vi "NHRDCPower.vi"() -> ()   [LabVIEW 2018, in "Visualization.lvlib" / "VisualizeAcPwr.lvclass"]
doc: "This VI listens for any measurement data associated with the provided PluginName and displays it to the user for analysis. The display is only suitable for data coming from the RoomAlert Plugin."
uses:
  VisualizeAcPwr.lvclass
  ChromaPowerSupply/Loop Parameters.ctl
  VisualizeBase/VisualizeBase_class/SubVIs/VisualizationOptions.ctl
  <vilib>/Utility/miscctls.llb/LVRectTypeDef.ctl
  AcPwr/AcPwrPlugins/NHRDCPowerClass/TypeDefs/Device(s)Settings.ctl
  AcPwr/AcPwrPlugins/NHRDCPowerClass/TypeDefs/Modules.ctl
  AcPwr/AcPwrPlugins/NHRDCPowerClass/TypeDefs/Measurements.ctl
  AcPwr/AcPwrShared/clMeasurmentData.ctl
  AcPwr/AcPwrPlugins/AcPwrBaseClass/TypeDefs/SetParameterInputs.ctl
  <vilib>/event_ctls.llb/usereventprio.ctl
  VisualizeBase/VisualizeBase_class/Requests/VisUserEventType.ctl
  <vilib>/Utility/error.llb/Error Cluster From Error Code.vi
  <vilib>/ErrorRing/Error Ring.xnode
  <userlib>/NIST/NISTErrorLib/NISTErrorLib.lvlib
  VisualizeBase/VisualizeBase_class/VisualizeBase.lvclass
  TestClass/Test.lvclass
  Sensor/VisualizeSensor.lvclass
  StatusAndLog/VisualizeStatus.lvclass
  AcPwr/AcPwrShared/AcPwrShared.lvlib
  AcPwr/AcPwrModule/AcPwrModule.lvlib
  AcPwr/AcPwrPlugins/AcPwrPlugins.lvlib
  AcPwr/AcPwrPlugins/AcPwrBaseClass/AcPwrBase.lvclass
  AcPwr/AcPwrPlugins/NHRDCPowerClass/NHRDCPower.lvclass
panel:
  out "Chart#":i32
  out "MeasChannels":string[](array[string])
  out "Writetime":u32 caption="Sample Write Time(ms)"
  out "ExitHelperLoops?":bool
  in  "Display":enum16{"Raw Data", "Voltage Vs Current"}(ring)
  in  "btnPause":bool
  in  "INIFilePath":path
  in  "ModuleID":i32
  in  "Log Data":bool=TRUE
  in  "btnStop":bool
  in  "btnReset":bool
  in  "btnClearTest":bool
  in  "btnStopModule":bool
  out "XY Graph":cluster{dbl[], dbl[]}(graph)
  out "Chart":waveform(dbl)[](graph)=[{"t0"=timestamp(3657200531.6397257 s since 1904-01-01), "dt"=1.0, "Y"=[46.19]}, {"t0"=timestamp(3657200531.6397257 s since 1904-01-01), "dt"=1.0, "Y"=[2.0]}, {"t0"=timestamp(3657200531.6397257 s since 1904-01-01), "dt"=1.0, "Y"=[60.0]}]
  in  "Power":bool
  in  "Power (W)":dbl
  in  "btnP_enable":bool
  in  "btnR_enable":bool
  in  "Resistance":bool
  in  "Resistance (Ohm)":dbl
  in  "btnI_enable":bool
  in  "Current":bool
  in  "Current (A)":dbl
  in  "btnV_Enable":bool
  in  "Voltage":bool
  in  "Voltage (V)":dbl
  in  "btnStopParameterLoop":bool
  in  "btnRunParamLoop":bool
  in  "Loop Parameters":T1={"Parameter"=enum."Voltage", "Start Value"=5.0, "Increment"=1.0, "Interval (s)"=3.0, "# Iterations"=6, "End Value"=10.0} {"# Iterations" min=1; "Increment" format="%#.4f"}
  out "ErrorArray":errorcluster[](array[cluster])
  out "Incorrect DataType?":bool
  out "String Results":string
  in  "PluginName":string="Sensor.RoomAlert1"
  # "Set Parameter"
  # "Parameter Looping"
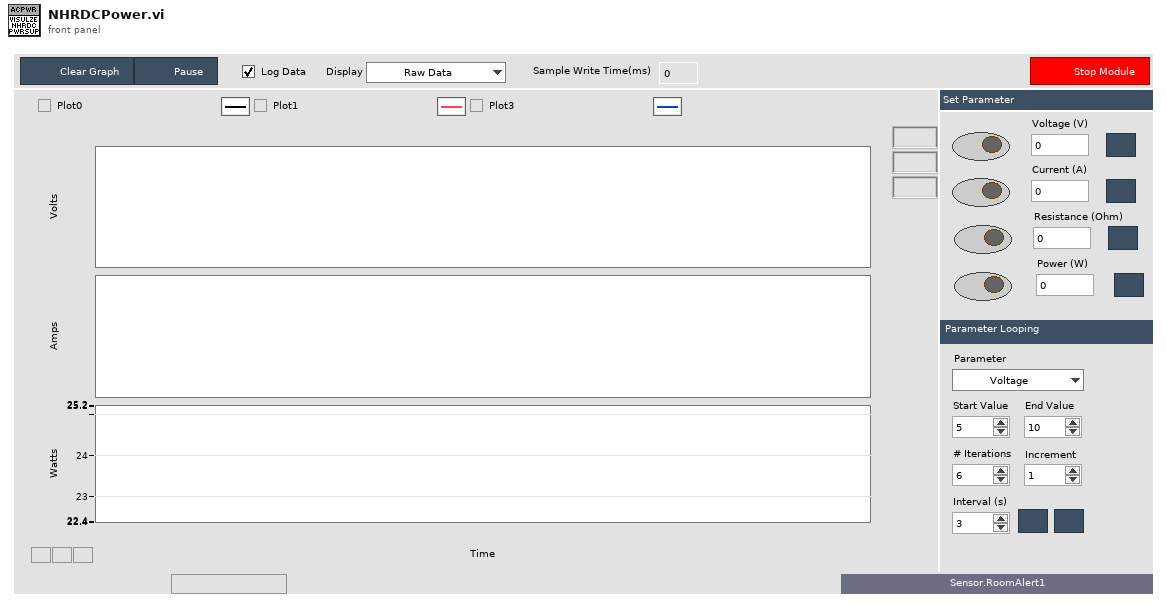
[diagram p1: front panel]
types:
  T1 = typedef "Loop Parameters.ctl" = cluster{"Parameter":enum16{"Voltage", "Current", "Power", "Resistance"}, "Start Value":dbl, "Increment":dbl, "Interval (s)":dbl, "# Iterations":u32, "End Value":dbl}
  T2 = typedef "Visualization.lvlib/VisualizeBase.lvclass/VisualizationOptions.ctl" = cluster{"PauseAtStartup":bool, "LogData":bool, "LaunchInSubPanel":bool, "FPMonitor":u16, "FPWindowBounds":T3, "MonitorBounds":cluster{"Left":i16, "Top":i16, "Right":i16, "Bottom":i16}, "MeasIndices":i32[]}
  T3 = typedef "LVRectTypeDef.ctl" = cluster{"Left":i16, "Top":i16, "Right":i16, "Bottom":i16}
  T4 = enum16{"open", "open or create", "create or replace", "create", "open (read-only)"}
  T5 = typedef "Visualization.lvlib/VisualizeBase.lvclass/VisRequestEvents.ctl" = cluster{"StopRequest":refnum<user-event>, "ResetRequest":refnum<user-event>, "FP Pop In or Out":refnum<user-event>}
  T6 = typedef "AcPwrShared.lvlib/AcPwrBroadcastEvents.ctl" = cluster{"DidInit":refnum<user-event>, "StatusUpdate":refnum<user-event>, "ErrorReport":refnum<user-event>, "DidStop":refnum<user-event>, "PathToINI":refnum<user-event>, "Measurements":refnum<user-event>, "LoadConfigFile":refnum<user-event>, "GetSettings":refnum<user-event>, "SetSettings":refnum<user-event>, "GetType&ID":refnum<user-event>, "GotSettings":refnum<user-event>, "GotSettingsLV":refnum<user-event>, "ParameterSet":refnum<user-event>}
  T7 = typedef "Visualization.lvlib/VisualizeBase.lvclass/VisFrmWrkBroadcastEvents.ctl" = cluster{"StatusUpdate":refnum<user-event>, "DidStop":refnum<user-event>, "NewModuleLoaded":refnum<user-event>, "StopVisualization":refnum<user-event>}
  T8 = typedef "AcPwrPlugins.lvlib/NHRDCPower.lvclass/Device(s)Settings.ctl" = cluster{"MeasName":string, "Modules":T9}
  T9 = typedef "AcPwrPlugins.lvlib/NHRDCPower.lvclass/Modules.ctl" = cluster{"Handle":string, "Name":string, "id query (Yes)":bool, "reset device (Yes)":bool, "Connected":bool, "Initial Battery Detect Voltage (0)":dbl, "SafetySettings":cluster{"SetWatchDog?":bool, "Voltage (V)":dbl, "Current (A)":dbl, "Power (W)":dbl, "Voltage Delay (s)":dbl, "Current Delay (s)":dbl, "Power Delay (s)":dbl}, "Options String":string, "Aperture Time (s)":dbl, "operating state (Off)":i32, "OutputSettings":cluster{"Voltage (V)":dbl, "Current (A)":dbl, "Resistance (Ohms)":dbl, "Power (W)":dbl, "Enable Voltage":bool, "Enable Current":bool, "Enable Resistance":bool, "Enable Power":bool, "Macro After Step Delay  (s)":dbl, "Wait Value (V, A, W)":dbl, "Enable Wait":bool, "Wait on Value":i32}[], "SlewRate":cluster{"Set Voltage Rate V/S":dbl, "Set Current Rate A/S":dbl, "Set Resistance Rate R/S":dbl, "Set Power Rate W/S":dbl}, "Macro":cluster{"Save Macro?":bool, "Load Macro From File?":bool, "Run Macro Continuously?":bool, "Use Macros?":bool, "Load Macro File Path":string, "Save Macro File Path":string}, "Regulation Gain (1=100%)":dbl, "UpdatingOntheFly":bool}[]
  T10 = typedef "AcPwrPlugins.lvlib/NHRDCPower.lvclass/Measurements.ctl" = cluster{"Handle":string, "Name":string, "Enabled":bool, "Measurement Value":sgl, "Measurement Type":enum16{"Power", "Current", "Voltage"}}[]
  T11 = typedef "AcPwrShared.lvlib/clMeasurmentData.ctl" = cluster{"MeasName":string, "XML Data":string, "WaveformData":waveform(dbl)[]}
  T12 = typedef "AcPwrPlugins.lvlib/AcPwrBase.lvclass/SetParameterInputs.ctl" = cluster{"Type":string, "Parameter":string, "Phase":i32, "Value":dbl, "Command":string, "Time Stamp":timestamp}
  T13 = typedef "Visualization.lvlib/VisualizeBase.lvclass/VisUserEventType.ctl" = cluster{"BusIndex":i8, "Data":variant}
  T14 = typedef "usereventprio.ctl" = enum32{"high priority", "normal priority"}
  T15 = cluster{"Handle":string, "Name":string, "id query (Yes)":bool, "reset device (Yes)":bool, "Connected":bool, "Initial Battery Detect Voltage (0)":dbl, "SafetySettings":cluster{"SetWatchDog?":bool, "Voltage (V)":dbl, "Current (A)":dbl, "Power (W)":dbl, "Voltage Delay (s)":dbl, "Current Delay (s)":dbl, "Power Delay (s)":dbl}, "Options String":string, "Aperture Time (s)":dbl, "operating state (Off)":i32, "OutputSettings":cluster{"Voltage (V)":dbl, "Current (A)":dbl, "Resistance (Ohms)":dbl, "Power (W)":dbl, "Enable Voltage":bool, "Enable Current":bool, "Enable Resistance":bool, "Enable Power":bool, "Macro After Step Delay  (s)":dbl, "Wait Value (V, A, W)":dbl, "Enable Wait":bool, "Wait on Value":i32}[], "SlewRate":cluster{"Set Voltage Rate V/S":dbl, "Set Current Rate A/S":dbl, "Set Resistance Rate R/S":dbl, "Set Power Rate W/S":dbl}, "Macro":cluster{"Save Macro?":bool, "Load Macro From File?":bool, "Run Macro Continuously?":bool, "Use Macros?":bool, "Load Macro File Path":string, "Save Macro File Path":string}, "Regulation Gain (1=100%)":dbl, "UpdatingOntheFly":bool}
  T16 = cluster{"Voltage (V)":dbl, "Current (A)":dbl, "Resistance (Ohms)":dbl, "Power (W)":dbl, "Enable Voltage":bool, "Enable Current":bool, "Enable Resistance":bool, "Enable Power":bool, "Macro After Step Delay  (s)":dbl, "Wait Value (V, A, W)":dbl, "Enable Wait":bool, "Wait on Value":i32}[]
  T17 = cluster{"Voltage (V)":dbl, "Current (A)":dbl, "Resistance (Ohms)":dbl, "Power (W)":dbl, "Enable Voltage":bool, "Enable Current":bool, "Enable Resistance":bool, "Enable Power":bool, "Macro After Step Delay  (s)":dbl, "Wait Value (V, A, W)":dbl, "Enable Wait":bool, "Wait on Value":i32}
  T18 = cluster{"Voltage (V)":dbl, "Current (A)":dbl, "Resistance (Ohm)":dbl, "Power (W)":dbl, "btnV_Enable":bool, "btnI_enable":bool, "btnR_enable":bool, "btnP_enable":bool}
  T19 = typedef "sizeaction.ctl" = enum32{"Minimized", "Maximized", "Resized"}
  T20 = typedef "LVPoint32TypeDef.ctl" = cluster{"Horizontal":i32, "Vertical":i32}
  T21 = enum16{"Voltage", "Current", "Power", "Resistance"}
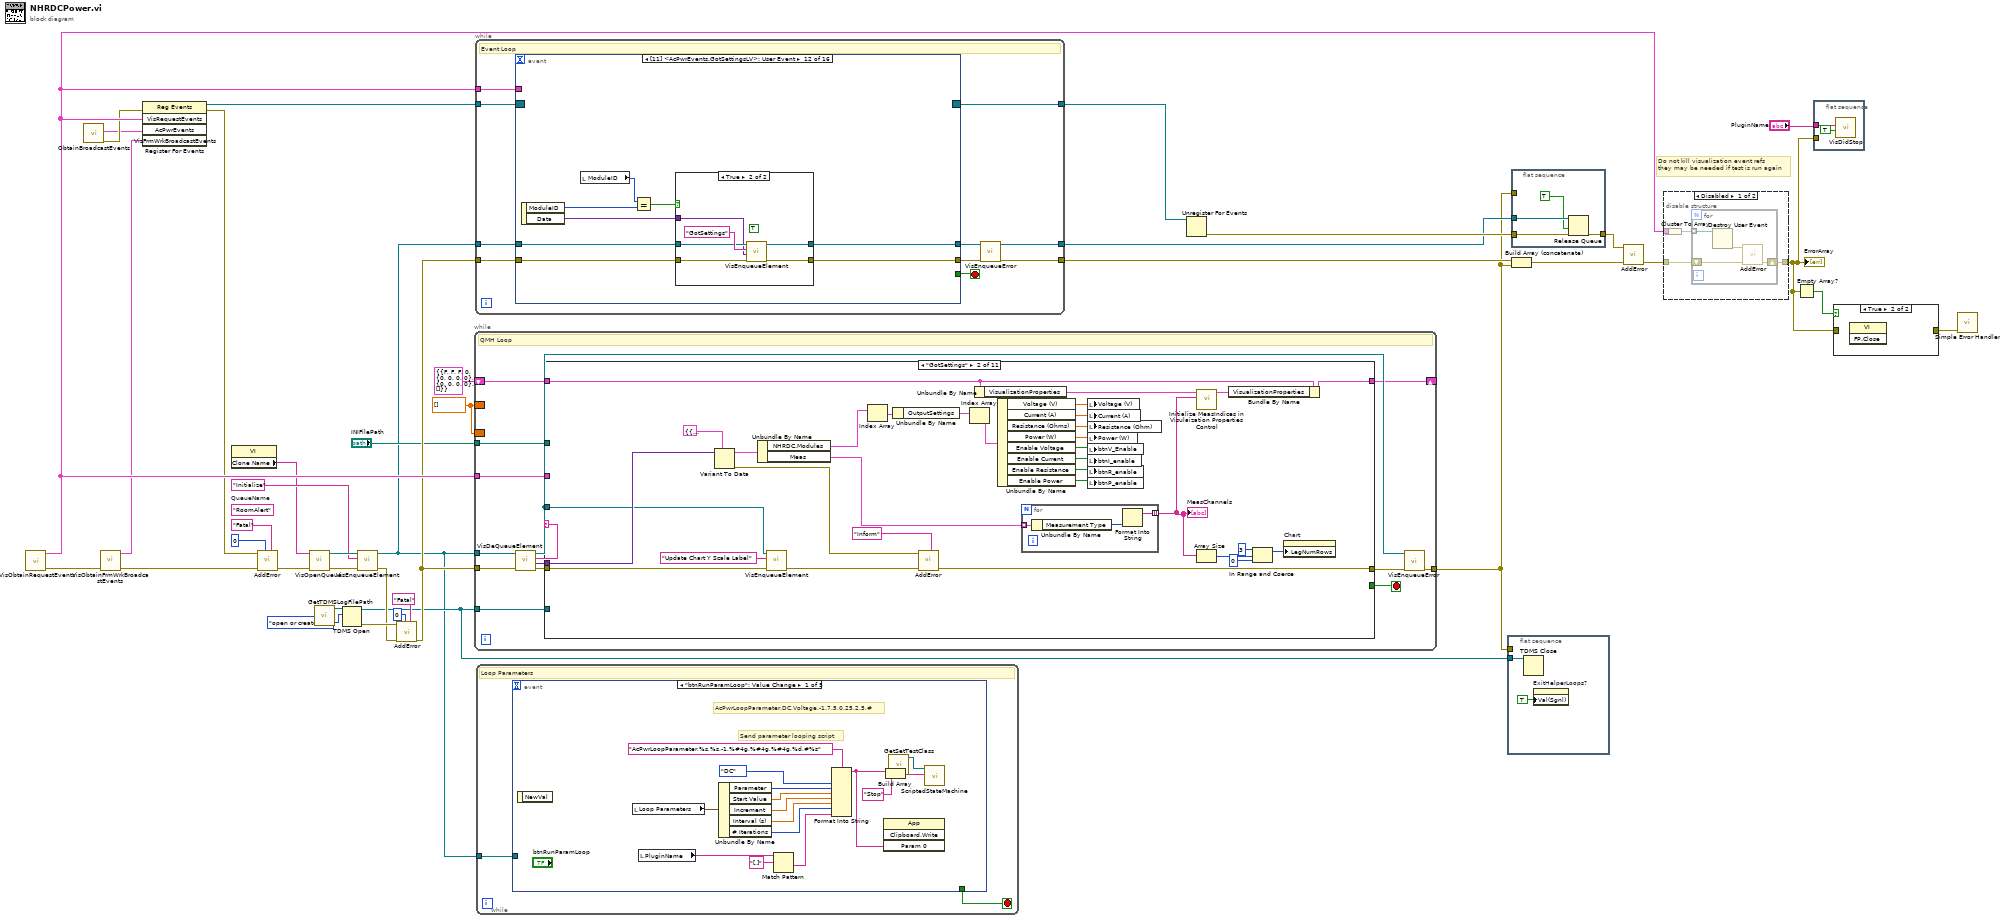
[diagram p0: block diagram]
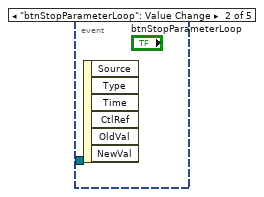
[diagram p2: hidden frame]
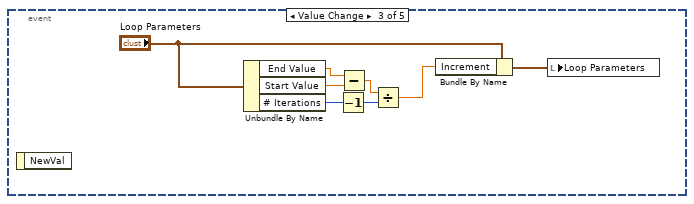
[diagram p3: hidden frame]
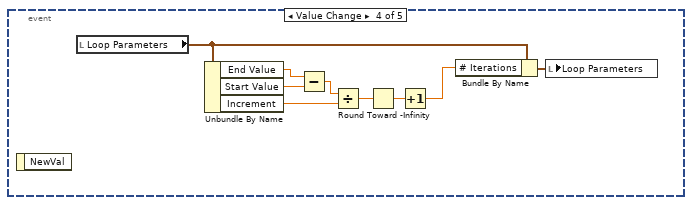
[diagram p4: hidden frame]
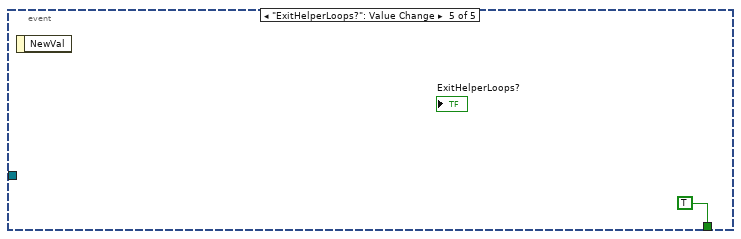
[diagram p5: hidden frame]
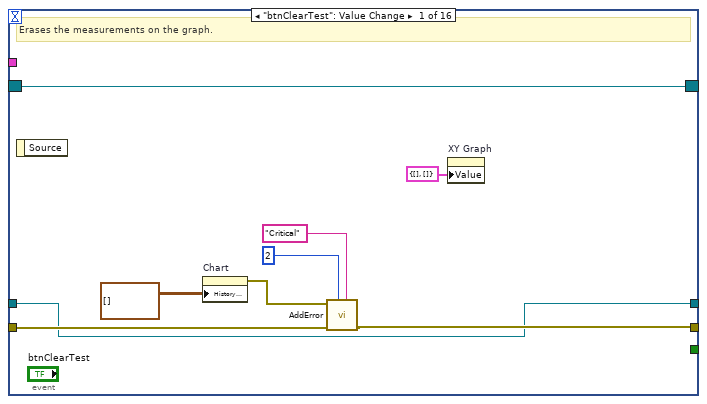
[diagram p7: hidden frame]
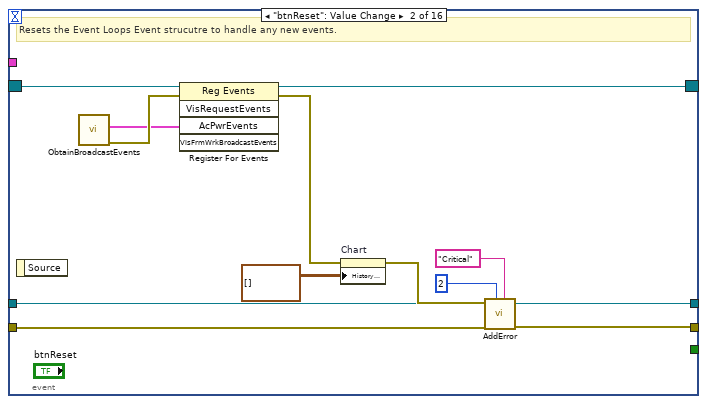
[diagram p8: hidden frame]
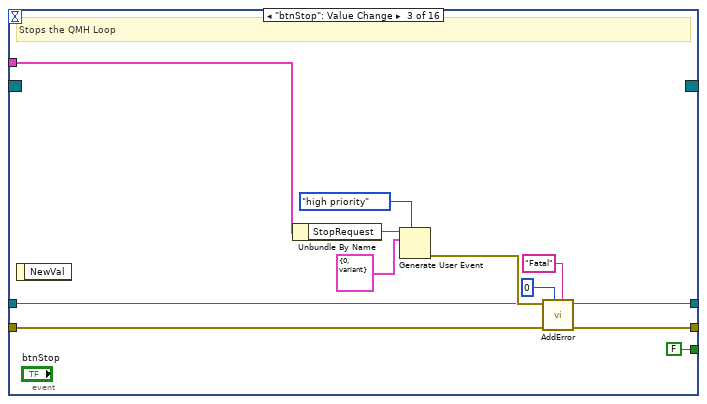
[diagram p9: hidden frame]
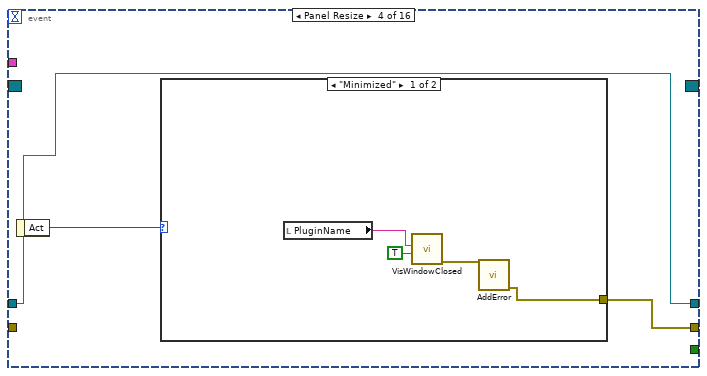
[diagram p10: hidden frame]
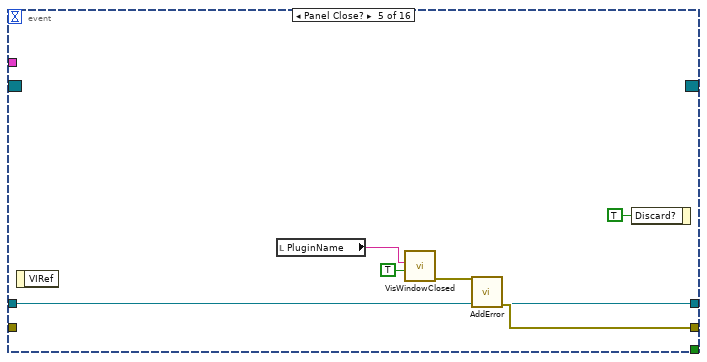
[diagram p12: hidden frame]
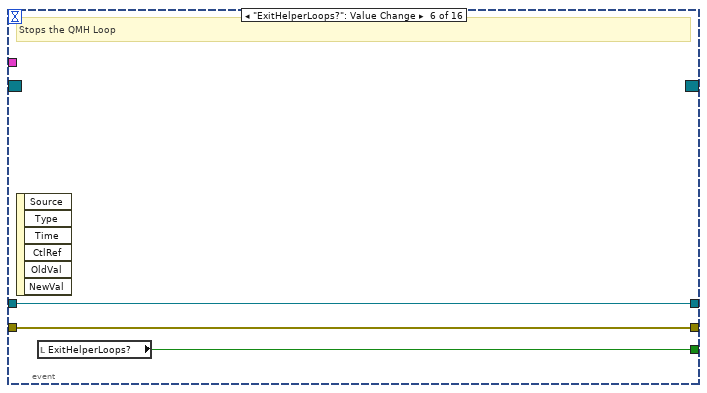
[diagram p13: hidden frame]
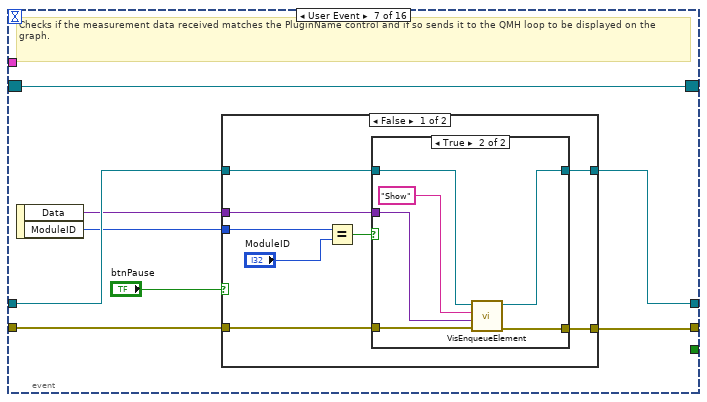
[diagram p14: hidden frame]
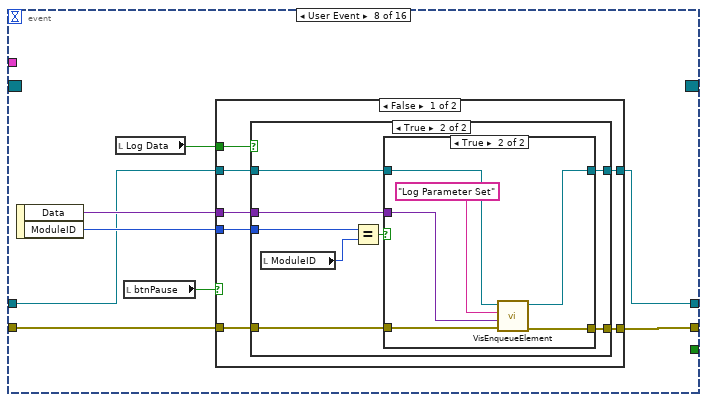
[diagram p17: hidden frame]
diagram:
  w2 = dbl[] []
  (unwired) "RoomAlert"  # QueueName
  # "Do not kill visualization event refs\nthey may be needed if test is run again"
  n1 = call "VisObtainRequestEvents.vi"() -> ("Error"=w30:errorcluster[], "VisRequestEvents"=w32:T5)  [unwired: 10 in]
  n2 = call "ObtainBroadcastEvents.vi"() -> ("error out"=w26:errorcluster, "AcPwrEvents"=w19:T6)  [unwired: 10 in]
  n3 = call "VisObtainFrmWrkBroadcastEvents.vi"("Error"=w30) -> ("Error"=w5:errorcluster[], "VisFrmWrkBroadcastEvents"=w4:T7)  [unwired: 9 in]
  n4 = register-events(error in=w26, w32, w19, w4) -> (reference out=w39:refnum<event-registration>, error out=w29:errorcluster)  [unwired: 1 in]
  n5 = property class="VI"() -> ("Clone Name"=w18:string)  [unwired: 2 in, 2 out]
  n6 = call <userlib>:"AddError.vi"("Severity"="Fatal", "Priority"=u8 0, "ErrorArray In"=w5, "error in (no error)"=w29) -> ("ErrorArray Out"=w25:errorcluster[])  [unwired: 6 in, 1 out]
  n7 = call "VisOpenQueue.vi"("Error Array In"=w25, "QueueName"=w18) -> ("Error Array Out"=w23:errorcluster[], "queue out"=w24:refnum<queue>)  [unwired: 8 in]
  n8 = call "GetTDMSLogFilePath.vi"() -> ("TDMS Log File Path"=w17:path)  [unwired: 11 in]
  n9 = TDMS Open(10:T4."open or create" ("operation (0:open)"), 11:w17) -> (0:w14:errorcluster, 3:w10:refnum<k34>)  [unwired: 5 in]
  n10 = call "VisEnqueueElement.vi"("Error Array In"=w23, "Message"="Initialize", "queue in"=w24) -> ("Error Array Out"=w13:errorcluster[], "queue out"=w3:refnum<queue>)  [unwired: 7 in]
  n11 = call <userlib>:"AddError.vi"("Severity"="Fatal", "Priority"=u8 0, "ErrorArray In"=w13, "error in (no error)"=w14) -> ("ErrorArray Out"=w12:errorcluster[])  [unwired: 6 in, 1 out]
  n12 = while {
    tunnel: w12 -> [w47]
    tunnel: [w50] -> w9
    tunnel: w3 -> [w46]
    tunnel: w32 -> [w52]
    tunnel: w10 -> [w43]
    tunnel: "INIFilePath" -> [w42]
    border: w2 -> [_]
    border: w2 -> [_]
    shift-right: [w40] -> _
    shift-left: cluster{"VisualizationProperties":T2} {"VisualizationProperties"={"PauseAtStartup"=FALSE, "LogData"=FALSE, "LaunchInSubPanel"=FALSE, "FPMonitor"=0, "FPWindowBounds"={"Left"=0, "Top"=0, "Right"=0, "Bottom"=0}, "MonitorBounds"={"Left"=0, "Top"=0, "Right"=0, "Bottom"=0}, "MeasIndices"=[]}} ("output cluster") -> [w41]
    stop <- w53 stop-if-true
    # "QMH Loop"
    n13 = call "VisDeQueueElement.vi"("Error Array In"=w47, "Queue In"=w46) -> ("Error Array Out"=w45:errorcluster[], "Data"=w48:variant, "Message"=w49:string, "Queue Out"=w44:refnum<queue>)  [unwired: 6 in]
    n14 = case shown="\"GotSettings\"" w49 {
      selector: w49 -> [_ _ _ _ _ _ w234 _ _ _ _]
      tunnel: w48 -> [_ w98 _ w119 w135 w209 _ w254 _ _ w312]
      tunnel: w45 -> [w66 w81 _ w116 w136 _ w232 _ w284 _ w308]
      tunnel: [w60 w97 _ w115 w137 _ w231 w244 w283 _ w310] -> w51
      tunnel: [_ _ _ _ _ _ _ w250 TRUE _ _] -> w53
      tunnel: w52 -> [_ _ _ _ _ _ _ w249 _ _ _]
      tunnel: w44 -> [_ w83 _ w117 _ _ _ w248 _ _ _]
      tunnel: w43 -> [_ _ _ _ w134 w208 _ _ _ _ _]
      tunnel: w42 -> [w65 _ _ _ _ _ _ _ w285 _ _]
      tunnel: w41 -> [w56 w89 w106 w126 w127 w206 w227 w242 w282 w289 w304]
      tunnel: [w55 w88 w106 w125 w127 w206 w227 w242 w282 w289 w304] -> w40
      frame "Initialize" {
        n15 = property on="Chart" class="WFChart (strict)"("History Data"=waveform(dbl)[][] []) -> ()  [unwired: 2 in, 2 out]
        n16 = property on="XY Graph" class="XYGraph (strict)"("Value"=cluster{dbl[], dbl[]} {[], []} ("XY Graph")) -> ()  [unwired: 2 in, 2 out]
        n17 = call "ApplyVisOptions.vi"("INIFilePath"=w65) -> ("error out"=w69:errorcluster, "VisualizationProperties"=w54:T2)  [unwired: 9 in]
        n18 = Bundle By Name(cluster=w56, "VisualizationProperties"=w54) -> (w55:cluster{"VisualizationProperties":T2})
        n19 = call <userlib>:"AddError.vi"("Severity"="Inform", "ErrorArray In"=w66, "error in (no error)"=w69) -> ("ErrorArray Out"=w67:errorcluster[])  [unwired: 7 in, 1 out]
        n20 = property on="Display" class="Enum (strict)"("Val(Sgnl)"="Display") -> ()  [unwired: 2 in, 2 out]
        n21 = local read "ModuleID"() -> (w57:i32)
        n22 = call "GetSettingsRequestLV.vi"("SettingsToGet"=variant, "ModuleID"=w57) -> ("Error Out"=w59:errorcluster)  [unwired: 9 in]
        n23 = call <userlib>:"AddError.vi"("Severity"="Inform", "ErrorArray In"=w67, "error in (no error)"=w59) -> ("ErrorArray Out"=w60:errorcluster[])  [unwired: 7 in, 1 out]
      }
      frame "GotSettings" {
        n24 = Variant To Data(type=cluster{"NHRDC":T8, "Meas":T10} {"NHRDC"={"MeasName"="", "Modules"=[]}, "Meas"=[]} ("output cluster"), Variant=w98) -> (data=w99:cluster{"NHRDC":T8, "Meas":T10}, error out=w96:errorcluster)  [unwired: 1 in]
        n25 = Unbundle By Name(w99) -> ("NHRDC.Modules"=w100:T9, "Meas"=w91:T10)
        n26 = call "VisEnqueueElement.vi"("Error Array In"=w81, "Message"="Update Chart Y Scale Label", "queue in"=w83) -> ("Error Array Out"=w82:errorcluster[])  [unwired: 7 in, 1 out]
        n27 = Index Array(array=w100) -> (element=w101:T15)  [unwired: 1 in]
        n28 = Unbundle By Name(w101) -> ("OutputSettings"=w80:T16)
        n29 = call <userlib>:"AddError.vi"("Severity"="Inform", "ErrorArray In"=w82, "error in (no error)"=w96) -> ("ErrorArray Out"=w97:errorcluster[])  [unwired: 7 in, 1 out]
        n30 = Index Array(array=w80) -> (element=w78:T17)  [unwired: 1 in]
        n31 = Unbundle By Name(w89) -> ("VisualizationProperties"=w86:T2)
        n32 = Unbundle By Name(w78) -> ("Voltage (V)"=w77:dbl, "Current (A)"=w76:dbl, "Resistance (Ohms)"=w75:dbl, "Power (W)"=w74:dbl, "Enable Voltage"=w73:bool, "Enable Current"=w72:bool, "Enable Resistance"=w71:bool, "Enable Power"=w70:bool)
        n33 = for {
          tunnel: w91 -> [w104] mode=indexing
          tunnel: [w102] -> w85 mode=indexing
          n34 = Unbundle By Name(w104) -> ("Measurement Type"=w103:enum16{"Power", "Current", "Voltage"})
          n35 = Format Into String(w103) -> (resulting string=w102:string)  [unwired: 3 in, 1 out]
        }
        "MeasChannels" <- w85
        n36 = local write "Voltage (V)"(w77) -> ()
        n37 = local write "Current (A)"(w76) -> ()
        n38 = local write "Resistance (Ohm)"(w75) -> ()
        n39 = local write "Power (W)"(w74) -> ()
        n40 = local write "btnV_Enable"(w73) -> ()
        n41 = local write "btnI_enable"(w72) -> ()
        n42 = local write "btnR_enable"(w71) -> ()
        n43 = local write "btnP_enable"(w70) -> ()
        n44 = call "Initialize MeasIndices in Visulaization Properties Control.vi"("MeasChannels"=w85, "VisualizationProperties"=w86) -> ("VisualizationProperties out"=w87:T2)  [unwired: 8 in, 1 out]
        n45 = Array Size(array=w85) -> (size(s)=w94:i32)
        n46 = Bundle By Name(cluster=w89, "VisualizationProperties"=w87) -> (w88:cluster{"VisualizationProperties":T2})
        n47 = In Range and Coerce(upper limit=3, x=w94, lower limit=0) -> (coerced(x)=w90:i32)  [unwired: 1 out]
        n48 = property on="Chart" class="WFChart (strict)"("LegNumRows"=w90) -> ()  [unwired: 2 in, 2 out]
      }
      frame "Update Chart Y Scale Label" {
        n49 = Unbundle By Name(w106) -> ("VisualizationProperties.MeasIndices"=w107:i32[])
        n50 = control-ref of="Chart"() -> (w109:refnum<vi>)
        n51 = local read "MeasChannels"() -> (w108:string[])
        n52 = for {
          tunnel: w107 -> [w112] mode=indexing
          tunnel: w109 -> [w114]
          tunnel: w108 -> [w113]
          i -> [w111]
          n53 = Index Array(array=w113, index=w112) -> (element=w110:string)
          n54 = property class="WFChart (strict)"(reference=w114, "ActYScl"=w111, "YScale.NameLbl.Text"=w110, "Active Plot"=w111, "Plot.Plot Name"=w110) -> ()  [unwired: 1 in, 2 out]
        }
        n55 = property on="Chart" class="WFChart (strict)"("History Data"=waveform(dbl)[][] []) -> ()  [unwired: 2 in, 2 out]
      }
      frame "Meas Variable Changed" {
        n56 = Unbundle By Name(w126) -> ("VisualizationProperties"=w124:T2)
        n57 = Variant To Data(type="" ("Message"), Variant=w119) -> (data=w118:string)  [unwired: 1 in, 1 out]
        n58 = local read "Chart#"() -> (w122:i32)
        n59 = call "Update MeasIndices in Visualization Properties Control.vi"("Item Tag"=w118, "Chart# user clicked on"=w122, "VisualizationProperties In"=w124) -> ("VisualizationProperties"=w123:T2)  [unwired: 8 in]
        n60 = Bundle By Name(cluster=w126, "VisualizationProperties"=w123) -> (w125:cluster{"VisualizationProperties":T2})
        n61 = call "VisEnqueueElement.vi"("Error Array In"=w116, "Message"="Update Chart Y Scale Label", "queue in"=w117) -> ("Error Array Out"=w115:errorcluster[])  [unwired: 7 in, 1 out]
      }
      frame "Show" {
        n62 = flat-sequence {
          tunnel: w134 -> [w139]
          tunnel: w135 -> [w140]
          tunnel: w136 -> [w141]
          tunnel: [w141] -> w133
          tunnel: [w140] -> w132
          tunnel: [w139] -> w131
          tunnel: [w138] -> w130
          tunnel: w133 -> [w157]
          tunnel: w132 -> [w156]
          tunnel: w131 -> [w151]
          tunnel: w130 -> [w144]
          tunnel: [w158] -> w129
          tunnel: [w144] -> w128
          tunnel: w127 -> [w143]
          tunnel: [w205] -> w137
          tunnel: w129 -> [w205]
          tunnel: w128 -> [w203]
          frame #0 {
            n63 = Tick Count (ms)() -> (millisecond timer value=w138:u32)
          }
          frame #1 {
            w153 = u32[] [0, 1, 2]  # PlotYAxis
            n64 = Variant To Data(type=T11 {"MeasName"="", "XML Data"="", "WaveformData"=[]} ("MeasurmentDataCluster"), Variant=w156) -> (data=w154:T11, error out=w155:errorcluster)  [unwired: 1 in]
            n65 = Unbundle By Name(w143) -> ("VisualizationProperties.MeasIndices"=w142:i32[])
            n66 = control-ref of="Chart"() -> (w145:refnum<vi>)
            n67 = Unbundle By Name(w154) -> ("WaveformData"=w146:waveform(dbl)[])
            n68 = call "RetrieveAcPwrMeasurementData.vi"("WaveformChartReference"=w145, "PlotYScale"=w153, "WaveformArrayIn"=w146, "error in (no error)"=w155) -> ("WaveformArrayOut"=w148:waveform(dbl)[], "OutputString(Chroma)"=w150:string, "Incorrect DataType?"=w149:bool, "error out"=w152:errorcluster)  [unwired: 7 in, 1 out]
            n69 = case shown="False" w149 {
              selector: w149 -> [w173 _]
              tunnel: [w182 w201] -> w158
              tunnel: w157 -> [w181 w201]
              tunnel: w152 -> [w178 _]
              tunnel: w151 -> [w175 _]
              tunnel: w150 -> [w174 _]
              tunnel: w148 -> [w161 _]
              tunnel: w142 -> [w159 _]
              frame False {
                n70 = for {
                  tunnel: w161 -> [w185]
                  tunnel: w159 -> [w184] mode=indexing
                  tunnel: [w183] -> w160 mode=indexing
                  n71 = Index Array(array=w185, index=w184) -> (element=w183:waveform(dbl))
                }
                "Chart" <- w160
                n72 = Index Array(array=w161, index #1=1 ("index"), index #2=0 ("index")) -> (element #1=w172:waveform(dbl), element #2=w171:waveform(dbl))
                n73 = Unbundle By Name(w172) -> ("Y"=w170:dbl[])
                n74 = Unbundle By Name(w171) -> ("Y"=w167:dbl[])
                n75 = feedback #1() -> (w169:dbl[])
                n76 = Build Array (concatenate)(w169, w170) -> (w164:dbl[])
                n77 = feedback-in #1(w164) -> ()
                n78 = feedback #2() -> (w168:dbl[])
                n79 = Build Array (concatenate)(w168, w167) -> (w163:dbl[])
                n80 = feedback-in #2(w163) -> ()
                n81 = Bundle(w164, w163) -> (→"XY Graph":cluster{dbl[], dbl[]})  [unwired: 1 in]
                n82 = case shown="True" "Log Data" {
                  tunnel: w178 -> [w186 w199]
                  tunnel: [w186 w200] -> w177
                  tunnel: w161 -> [_ w198]
                  tunnel: w175 -> [_ w193]
                  frame False {
                  }
                  frame True {
                    n83 = call "PrepareWaveformDataForTDMS.vi"("error in (no error)"=w199, "WaveformArray in"=w198) -> ("error out"=w197:errorcluster, "Measurement Data"=w195:dbl[][], "Channel Names"=w196:string[], "TimeStamp"=w188:timestamp)  [unwired: 6 in]
                    n84 = local read "PluginName"() -> (w191:string)
                    n85 = Build Array(w188) -> (w187:timestamp[])
                    n86 = TDMS Write(0:w193, 5:w191, 7:"TimeStamp" ("PluginName"), 9:w187, 11:w197) -> (4:w192:refnum<k34>, 6:w190:string, 15:w194:errorcluster)  [unwired: 1 in, 1 out]
                    n87 = TDMS Write(0:w192, 5:w190, 7:w196, 9:w195, 11:w194) -> (15:w200:errorcluster)  [unwired: 1 in, 3 out]
                  }
                }
                n88 = call <userlib>:"AddError.vi"("Severity"="Fatal" ("String"), "Priority"=u8 0, "ErrorArray In"=w181, "error in (no error)"=w177) -> ("ErrorArray Out"=w182:errorcluster[])  [unwired: 6 in, 1 out]
                "String Results" <- w174
                "Incorrect DataType?" <- w173
              }
              frame True {
              }
            }
          }
          frame #2 {
            n89 = Tick Count (ms)() -> (millisecond timer value=w204:u32)
            n90 = Subtract(x=w204, y=w203) -> (x-y=→"Writetime":u32)
          }
        }
      }
      frame "Log Parameter Set" {
        n91 = Variant To Data(type=T12 {"Type"="", "Parameter"="", "Phase"=0, "Value"=0.0, "Command"="", "Time Stamp"=timestamp(0 s since 1904-01-01)}, Variant=w209) -> (data=w221:T12, error out=w210:errorcluster)  [unwired: 1 in]
        n92 = Unbundle By Name(w221) -> ("Type"=w220:string, "Parameter"=w219:string, "Phase"=w218:i32, "Time Stamp"=w214:timestamp, "Value"=w212:dbl)
        n93 = local read "PluginName"() -> (w207:string)
        n94 = Format Into String(format string="Set-%s_%s_Phase_%d", w220, w219, w218) -> (resulting string=w213:string)  [unwired: 2 in, 1 out]
        n95 = Concatenate Strings(w213, "_TimeStamp" ("string")) -> (w215:string)
        n96 = Build Array(w214) -> (w222:timestamp[])
        n97 = Build Array(w212) -> (w211:dbl[])
        n98 = TDMS Write(0:w208, 5:w207, 7:w215, 9:w222, 11:w210) -> (4:w224:refnum<k34>, 6:w223:string, 15:w225:errorcluster)  [unwired: 1 in, 1 out]
        n99 = TDMS Write(0:w224, 5:w223, 7:w213, 9:w211, 11:w225) -> ()  [unwired: 1 in, 4 out]
      }
      frame Default {
        n100 = xnode "Error Ring"("parameter 0"=w234) -> ("error out"=w233:errorcluster)
        n101 = call <userlib>:"AddError.vi"("Severity"="Inform" ("String"), "Priority"=u8 5, "ErrorArray In"=w232, "error in (no error)"=w233) -> ("ErrorArray Out"=w231:errorcluster[], "error out"=w230:errorcluster)  [unwired: 6 in]
        n102 = call <vilib>:"Clear Errors.vi"("error in (no error)"=w230) -> ()  [unwired: 5 in, 2 out]
      }
      frame "Error" {
        n103 = Variant To Data(type=errorcluster[] [], Variant=w254) -> (data=w252:errorcluster[], error out=w243:errorcluster)  [unwired: 1 in]
        n104 = call <userlib>:"ParseErrors.vi"("ErrorArray"=w252) -> ("ErrorArray"=w251:errorcluster[])  [unwired: 8 in, 2 out]
        n105 = for {
          tunnel: w251 -> [w265] mode=indexing
          tunnel: [w259] -> w245 mode=concatenating
          tunnel: [w257] -> w250
          tunnel: w249 -> [w256]
          tunnel: w248 -> [w255]
          stop <- w257 stop-if-true
          n106 = call <userlib>:"GeneralHandler.vi"("error in (no error)"=w265) -> ("Severity"=w258:string, "Stop"=w262:bool, "Abort"=w263:bool, "Continue"=w264:bool)  [unwired: 6 in, 1 out]
          n107 = Build Array(w264, w263, w262) -> (w261:bool[])
          n108 = Boolean Array To Number(Boolean array=w261) -> (number=w260:u32)
          n109 = case shown="1" w260 {
            tunnel: [_ _ w270 w279] -> w259
            tunnel: w258 -> [_ _ _ w272]
            tunnel: [_ _ _ w274] -> w257
            tunnel: w256 -> [_ _ _ w273]
            tunnel: w255 -> [_ _ w266 _]
            frame 0, Default {
              # "No Dialog"
            }
            frame 1 {
              # "Continue"
            }
            frame 2 {
              # "Abort, Flush Queue"
              n110 = Flush Queue(queue=w266) -> (error out=w269:errorcluster)  [unwired: 1 in, 2 out]
              n111 = call <userlib>:"AddError.vi"("Severity"="Critical" ("String"), "Priority"=u8 1, "error in (no error)"=w269) -> ("ErrorArray Out"=w270:errorcluster[])  [unwired: 7 in, 1 out]
            }
            frame 4 {
              # "Stop"
              n112 = Unbundle By Name(w273) -> ("StopRequest"=w280:refnum<user-event>)
              n113 = Equal?(x=w272, y="Fatal" ("x")) -> (x = y?=w274:bool)
              n114 = Generate User Event(priority (normal)=usereventprio."high priority", user event=w280, event data cluster=T13 {"BusIndex"=0, "Data"=variant} ("event data")) -> (error out=w278:errorcluster)  [unwired: 1 in, 1 out]
              n115 = call <userlib>:"AddError.vi"("error in (no error)"=w278) -> ("ErrorArray Out"=w279:errorcluster[], "error out"=w275:errorcluster)  [unwired: 9 in]
              n116 = call <vilib>:"Clear Errors.vi"("error in (no error)"=w275) -> ()  [unwired: 5 in, 2 out]
            }
          }
        }
        n117 = call <userlib>:"AddError.vi"("Severity"="Critical", "Priority"=u8 2, "ErrorArray In"=w245, "error in (no error)"=w243) -> ("ErrorArray Out"=w244:errorcluster[])  [unwired: 6 in, 1 out]
      }
      frame "Stop" {
        n118 = Unbundle By Name(w282) -> ("VisualizationProperties"=w281:T2)
        n119 = call "WriteVisOptionsToINIFile.vi"("Visualization Options"=w281, "INIFilePath"=w285) -> ("error out"=w286:errorcluster)  [unwired: 8 in, 1 out]
        n120 = call <userlib>:"AddError.vi"("Severity"="Inform", "ErrorArray In"=w284, "error in (no error)"=w286) -> ("ErrorArray Out"=w283:errorcluster[])  [unwired: 7 in, 1 out]
      }
      frame "- ---AcPwr Module Specific Commands----" {
      }
      frame "Set Parameter" {
        n121 = Variant To Data(type="", Variant=w312) -> (error out=w309:errorcluster)  [unwired: 1 in, 1 out]
        n122 = call <userlib>:"AddError.vi"("Severity"="Inform", "Priority"=u8 0, "ErrorArray In"=w308, "error in (no error)"=w309) -> ("ErrorArray Out"=w305:errorcluster[])  [unwired: 6 in, 1 out]
        n123 = Bundle("Voltage (V)"="Voltage (V)", "Current (A)"="Current (A)", "Resistance (Ohm)"="Resistance (Ohm)", "Power (W)"="Power (W)", "btnV_Enable"="btnV_Enable", "btnI_enable"="btnI_enable", "btnR_enable"="btnR_enable", "btnP_enable"="btnP_enable") -> (w299:T18)  [unwired: 1 in]
        n124 = Flatten To XML(anything=w299) -> (xml string=w298:string)
        n125 = local read "PluginName"() -> (w317:string)
        n126 = Match Pattern(string=w317, regular expression="[.]") -> (after substring=w318:string)  [unwired: 1 in, 3 out]
        n127 = Format Into String(format string="AcPwrSetParameter,%s,%s,-1,%.4f,#%s", enum16{"AC", "DC"}."DC" ("input 1"), w298, 0.0 ("input 3"), w318) -> (resulting string=w316:string)  [unwired: 2 in, 1 out]
        n128 = call "GetSetTestClass.vi"() -> ("Test.lvclass"=w296:refnum<class "Test.lvclass">)  [unwired: 11 in]
        n129 = Build Array(w316, "Stop" ("element")) -> (w295:string[])
        n130 = call "ScriptedStateMachine.vi"("ErrorArray 2"=w305, "script"=w295, "Test.lvclass 2"=w296) -> ("ErrorArray"=w310:errorcluster[])  [unwired: 6 in, 2 out]
      }
    }
    n131 = call "VisEnqueueError.vi"("Error Array In"=w51, "Queue in"=w44) -> ("Error Array Out"=w50:errorcluster[])  [unwired: 8 in, 1 out]
  }
  n132 = while {
    tunnel: w39 -> [w328]
    tunnel: [w322] -> w37
    tunnel: [w326] -> w38
    tunnel: w32 -> [w325]
    tunnel: w12 -> [w324]
    tunnel: w3 -> [w323]
    tunnel: [w319] -> w21
    stop <- w327 stop-if-true
    # "Event Loop"
    n133 = event shown="[11] <AcPwrEvents.GotSettingsLV>: User Event" {
      selector: w328 -> [w331 w349 _ _ _ _ w380 _ _ _ _ _ _ _ _ _]
      dyn-events: [w331 w348 _ _ _ _ w380 _ _ _ _ _ _ _ _ _] -> w326
      timeout: _ -> [_ _ _ _ _ _ _ _ _ _ _ _ _ _ _ _]
      tunnel: [_ _ FALSE ("Priority? (F)") _ _ w374 _ _ _ _ _ _ _ _ _ _] -> w327
      tunnel: [w334 w346 w353 w362 w369 w375 w382 w403 w441 _ w463 w471 w482 w492 _ w515] -> w321
      tunnel: w325 -> [_ _ w352 _ _ _ _ _ _ _ _ _ _ _ _ _]
      tunnel: w324 -> [w335 w347 w360 _ _ w375 w383 w405 w440 _ _ w469 _ w491 _ w517]
      tunnel: w323 -> [w329 w339 w350 w361 w368 w376 w384 w406 w443 w453 w461 w468 w481 w494 _ w518]
      tunnel: [w329 w339 w350 w361 w368 w376 w381 w404 w442 w453 w462 w470 w481 w493 _ w516] -> w320
      event "btnClearTest": Value Change {
        # "Erases the measurements on the graph."
        n134 = event-data() -> ()  [unwired: 1 in, 1 out]
        n135 = property on="Chart" class="WFChart (strict)"("History Data"=waveform(dbl)[][] []) -> (error out=w333:errorcluster)  [unwired: 2 in, 1 out]
        n136 = call <userlib>:"AddError.vi"("Severity"="Critical", "Priority"=u8 2, "ErrorArray In"=w335, "error in (no error)"=w333) -> ("ErrorArray Out"=w334:errorcluster[])  [unwired: 6 in, 1 out]
        n137 = property on="XY Graph" class="XYGraph (strict)"("Value"=cluster{dbl[], dbl[]} {[], []} ("XY Graph")) -> ()  [unwired: 2 in, 2 out]
      }
      event "btnReset": Value Change {
        # "Resets the Event Loops Event strucutre to handle any new events."
        n138 = event-data() -> ()  [unwired: 1 in, 1 out]
        n139 = call "ObtainBroadcastEvents.vi"() -> ("error out"=w340:errorcluster, "AcPwrEvents"=w338:T6)  [unwired: 10 in]
        n140 = register-events(reference=w349, error in=w340, w338) -> (reference out=w348:refnum<event-registration>, error out=w342:errorcluster)  [unwired: 2 in]
        n141 = property on="Chart" class="WFChart (strict)"(error in=w342, "History Data"=waveform(dbl)[][] []) -> (error out=w341:errorcluster)  [unwired: 1 in, 1 out]
        n142 = call <userlib>:"AddError.vi"("Severity"="Critical", "Priority"=u8 2, "ErrorArray In"=w347, "error in (no error)"=w341) -> ("ErrorArray Out"=w346:errorcluster[])  [unwired: 6 in, 1 out]
      }
      event "btnStop": Value Change {
        # "Stops the QMH Loop"
        n143 = event-data() -> ()  [unwired: 1 in, 1 out]
        n144 = Unbundle By Name(w352) -> ("StopRequest"=w358:refnum<user-event>)
        n145 = Generate User Event(priority (normal)=usereventprio."high priority", user event=w358, event data cluster=T13 {"BusIndex"=0, "Data"=variant} ("event data")) -> (error out=w359:errorcluster)  [unwired: 1 in, 1 out]
        n146 = call <userlib>:"AddError.vi"("Severity"="Fatal" ("String"), "Priority"=u8 0, "ErrorArray In"=w360, "error in (no error)"=w359) -> ("ErrorArray Out"=w353:errorcluster[])  [unwired: 6 in, 1 out]
      }
      event Panel Resize {
        n147 = event-data() -> ("Act"=w363:T19)  [unwired: 1 in]
        n148 = case shown="\"Minimized\"" w363 {
          tunnel: [w364 _] -> w362
          frame "Minimized" {
            n149 = local read "PluginName"() -> (w366:string)
            n150 = call "VisWindowClosed.vi"("Window Closed?"=TRUE ("Window Minimized or Clozed?"), "Module Name"=w366) -> ("error out"=w367:errorcluster)  [unwired: 9 in]
            n151 = call <userlib>:"AddError.vi"("error in (no error)"=w367) -> ("ErrorArray Out"=w364:errorcluster[])  [unwired: 9 in, 1 out]
          }
          frame "Maximized", Default {
          }
        }
      }
      event Panel Close? {
        n152 = event-data() -> ()  [unwired: 1 in, 1 out]
        n153 = local read "PluginName"() -> (w370:string)
        n154 = call "VisWindowClosed.vi"("Window Closed?"=TRUE ("Window Minimized or Clozed?"), "Module Name"=w370) -> ("error out"=w371:errorcluster)  [unwired: 9 in]
        n155 = call <userlib>:"AddError.vi"("error in (no error)"=w371) -> ("ErrorArray Out"=w369:errorcluster[])  [unwired: 9 in, 1 out]
        n156 = event-data("Discard?"=TRUE) -> ()  [unwired: 1 in, 1 out]
      }
      event "ExitHelperLoops?": Value Change {
        # "Stops the QMH Loop"
        n157 = event-data() -> ()  [unwired: 1 in, 6 out]
        n158 = local read "ExitHelperLoops?"() -> (w374:bool)
      }
      event User Event {
        # "Checks if the measurement data received matches the PluginName control and if so sends it to the QMH loop to be displayed on the graph."
        n159 = event-data() -> ("Data"=w379:variant, "ModuleID"=w378:i32)  [unwired: 1 in]
        n160 = case shown="False" "btnPause" {
          tunnel: w384 -> [w392 w402]
          tunnel: w383 -> [w391 w401]
          tunnel: [w390 w401] -> w382
          tunnel: [w389 w402] -> w381
          tunnel: w379 -> [w388 _]
          tunnel: w378 -> [w385 _]
          frame False {
            n161 = Equal?(x=w385, y="ModuleID") -> (x = y?=w387:bool)
            n162 = case shown="True" w387 {
              tunnel: [w393 w399] -> w390
              tunnel: w392 -> [w394 w398]
              tunnel: w391 -> [w393 w400]
              tunnel: [w394 w396] -> w389
              tunnel: w388 -> [_ w397]
              frame False {
              }
              frame True {
                n163 = call "VisEnqueueElement.vi"("Error Array In"=w400, "Data"=w397, "Message"="Show", "queue in"=w398) -> ("Error Array Out"=w399:errorcluster[], "queue out"=w396:refnum<queue>)  [unwired: 6 in]
              }
            }
          }
          frame True {
          }
        }
      }
      event User Event {
        n164 = event-data() -> ("Data"=w408:variant, "ModuleID"=w407:i32)  [unwired: 1 in]
        n165 = local read "Log Data"() -> (w409:bool)
        n166 = local read "btnPause"() -> (w410:bool)
        n167 = case shown="False" w410 {
          tunnel: w406 -> [w417 w437]
          tunnel: w405 -> [w416 w436]
          tunnel: [w415 w436] -> w403
          tunnel: [w414 w437] -> w404
          tunnel: w408 -> [w413 _]
          tunnel: w407 -> [w412 _]
          tunnel: w409 -> [w411 _]
          frame False {
            n168 = case shown="True" w411 {
              tunnel: w417 -> [w419 w427]
              tunnel: w416 -> [w418 w426]
              tunnel: [w418 w425] -> w415
              tunnel: [w419 w424] -> w414
              tunnel: w413 -> [_ w423]
              tunnel: w412 -> [_ w421]
              frame False {
              }
              frame True {
                n169 = local read "ModuleID"() -> (w420:i32)
                n170 = Equal?(x=w421, y=w420) -> (x = y?=w422:bool)
                n171 = case shown="True" w422 {
                  tunnel: [w428 w434] -> w425
                  tunnel: w427 -> [w429 w433]
                  tunnel: w426 -> [w428 w435]
                  tunnel: [w429 w431] -> w424
                  tunnel: w423 -> [_ w432]
                  frame False {
                  }
                  frame True {
                    n172 = call "VisEnqueueElement.vi"("Error Array In"=w435, "Data"=w432, "Message"="Log Parameter Set", "queue in"=w433) -> ("Error Array Out"=w434:errorcluster[], "queue out"=w431:refnum<queue>)  [unwired: 6 in]
                  }
                }
              }
            }
          }
          frame True {
          }
        }
      }
      event User Event {
        n173 = event-data() -> ("ModuleID"=w439:i32)  [unwired: 1 in, 5 out]
        n174 = local read "ModuleID"() -> (w438:i32)
        n175 = Equal?(x=w438, y=w439) -> (x = y?=w444:bool)
        n176 = case shown="True" w444 {
          tunnel: [w445 w450] -> w441
          tunnel: [w446 w449] -> w442
          tunnel: w443 -> [w446 w448]
          tunnel: w440 -> [w445 w447]
          frame False {
          }
          frame True {
            n177 = call "VisEnqueueElement.vi"("Priority? (F)"=TRUE, "Error Array In"=w447, "Message"="Stop", "queue in"=w448) -> ("Error Array Out"=w450:errorcluster[], "queue out"=w449:refnum<queue>)  [unwired: 6 in]
          }
        }
      }
      event "Display": Value Change {
        n178 = event-data() -> ("NewVal"=w456:enum16{"Raw Data", "Voltage Vs Current"})  [unwired: 1 in]
        n179 = case shown="\"Raw Data\", Default" w456 {
          tunnel: [TRUE FALSE] -> w455
          frame "Raw Data", Default {
          }
          frame "Voltage Vs Current" {
          }
        }
        n180 = Not(x=w455) -> (.not. x?=w454:bool)
        n181 = property on="Chart" class="WFChart (strict)"("Visible"=w455) -> ()  [unwired: 2 in, 2 out]
        n182 = property on="XY Graph" class="XYGraph (strict)"("Visible"=w454) -> ()  [unwired: 2 in, 2 out]
      }
      event "Resistance", "Current", "Power", "Voltage": Value Change {
        n183 = event-data() -> ("CtlRef"=w464:refnum<vi>)  [unwired: 1 in]
        n184 = property class="Bool"(reference=w464) -> ("Label.Text"=w459:string)  [unwired: 1 in, 2 out]
        n185 = call "VisEnqueueElement.vi"("Data"=w459, "Message"="Set Parameter", "queue in"=w461) -> ("Error Array Out"=w463:errorcluster[], "queue out"=w462:refnum<queue>)  [unwired: 7 in]
      }
      event User Event {
        n186 = event-data() -> ("ModuleID"=w466:i32, "Data"=w465:variant)  [unwired: 1 in]
        n187 = local read "ModuleID"() -> (w467:i32)
        n188 = Equal?(x=w467, y=w466) -> (x = y?=w472:bool)
        n189 = case shown="True" w472 {
          tunnel: w468 -> [w473 w479]
          tunnel: w469 -> [w474 w478]
          tunnel: [w473 w477] -> w470
          tunnel: [w474 w476] -> w471
          tunnel: w465 -> [_ w475]
          frame False {
          }
          frame True {
            (unwired) TRUE ("Priority? (F)")
            n190 = call "VisEnqueueElement.vi"("Error Array In"=w478, "Data"=w475, "Message"="GotSettings", "queue in"=w479) -> ("Error Array Out"=w476:errorcluster[], "queue out"=w477:refnum<queue>)  [unwired: 6 in]
          }
        }
      }
      event "btnStopModule": Value Change {
        n191 = event-data() -> ()  [unwired: 1 in, 1 out]
        n192 = local read "ModuleID"() -> (w484:i32)
        n193 = call "StatusUpdateByModID.vi"("Status"="User requested module stop", "Accessors:Module ID"=w484) -> ("error out"=w485:errorcluster)  [unwired: 9 in]
        n194 = flat-sequence {
          tunnel: [w487] -> w482
          tunnel: w485 -> [_]
          frame #0 {
            n195 = local read "PluginName"() -> (w486:string)
            n196 = call "GetSetTestClass.vi"() -> ("Test.lvclass"=w488:refnum<class "Test.lvclass">)  [unwired: 11 in]
            n197 = call "StopModByName.vi"("Module Name"=w486, "Test.lvclass"=w488) -> ("ErrorArray Out"=w487:errorcluster[])  [unwired: 4 in, 5 out]
          }
        }
      }
      event User Event {
        # "Framework requested visualization stop"
        n198 = event-data() -> ("Data"=w489:variant)  [unwired: 1 in]
        n199 = local read "PluginName"() -> (w490:string)
        n200 = Variant To Data(type="" ("Message"), Variant=w489) -> (data=w500:string, error out=w498:errorcluster)  [unwired: 1 in]
        n201 = call <userlib>:"AddError.vi"("Severity"="Inform", "Priority"=u8 3, "ErrorArray In"=w491, "error in (no error)"=w498) -> ("ErrorArray Out"=w497:errorcluster[])  [unwired: 6 in, 1 out]
        n202 = Equal?(x=w490, y=w500) -> (x = y?=w499:bool)
        n203 = case shown="True" w499 {
          tunnel: w494 -> [w503 w507]
          tunnel: [w502 w506] -> w492
          tunnel: w497 -> [w502 w505]
          tunnel: [w503 w504] -> w493
          frame False {
          }
          frame True {
            n204 = call "VisEnqueueElement.vi"("Priority? (F)"=TRUE, "Error Array In"=w505, "Message"="Stop", "queue in"=w507) -> ("Error Array Out"=w506:errorcluster[], "queue out"=w504:refnum<queue>)  [unwired: 6 in]
          }
        }
      }
      event "Chart": Shortcut Menu Activation? {
        n205 = event-data() -> ("CtlRef"=w513:refnum<vi>, "MenuRef"=w512:refnum<k9>, "Coords"=w511:T20)  [unwired: 1 in]
        n206 = local read "MeasChannels"() -> (w510:string[])
        n207 = call "Handle Chart Menu Activation.vi"("Channel Names"=w510, "Coords"=w511, "MenuRef"=w512, "CtlRef"=w513) -> ("Channel Index"=→"Chart#":i32)  [unwired: 7 in]
        n208 = event-data() -> ()  [unwired: 2 in, 1 out]
      }
      event "Chart": Shortcut Menu Selection (User) {
        n209 = event-data() -> ("ItemTag"=w519:string)  [unwired: 1 in]
        n210 = Match Pattern(string=w519, regular expression="Meas_") -> (after substring=w521:string, offset past match=w520:i32)  [unwired: 1 in, 2 out]
        n211 = case shown="Default" w520 {
          tunnel: w518 -> [w527 w530]
          tunnel: w517 -> [w526 w529]
          tunnel: [w525 w530] -> w516
          tunnel: [w524 w529] -> w515
          tunnel: w521 -> [w523 _]
          frame Default {
            # "User selected a measurement variable\nin the Chart shortcut menu"
            n212 = call "VisEnqueueElement.vi"("Error Array In"=w526, "Data"=w523, "Message"="Meas Variable Changed", "queue in"=w527) -> ("Error Array Out"=w524:errorcluster[], "queue out"=w525:refnum<queue>)  [unwired: 6 in]
          }
          frame -1 {
          }
        }
      }
    }
    n213 = call "VisEnqueueError.vi"("Error Array In"=w321, "Queue in"=w320) -> ("Error Array Out"=w322:errorcluster[], "Queue out"=w319:refnum<queue>)  [unwired: 8 in]
  }
  n214 = while {
    tunnel: w3 -> [w531]
    stop <- w532 stop-if-true
    # "Loop Parameters"
    n215 = event shown="[0] \"btnRunParamLoop\": Value Change" {
      selector: _ -> [_ _ _ _ _]
      dyn-events: _ -> [_ _ _ _ _]
      timeout: _ -> [_ _ _ _ _]
      tunnel: [_ _ _ _ TRUE] -> w532
      tunnel: w531 -> [_ _ _ _ _]
      event "btnRunParamLoop": Value Change {
        # "AcPwrLoopParameter,DC,Voltage,-1,7.5,0.25,2,5,#"
        # "Send parameter looping script"
        n216 = event-data() -> ()  [unwired: 1 in, 1 out]
        n217 = local read "Loop Parameters"() -> (w535:T1)
        n218 = local read "PluginName"() -> (w534:string)
        n219 = Unbundle By Name(w535) -> ("Parameter"=w546:T21, "Start Value"=w545:dbl, "Increment"=w544:dbl, "Interval (s)"=w543:dbl, "# Iterations"=w542:u32)
        n220 = Match Pattern(string=w534, regular expression="[.]") -> (after substring=w537:string)  [unwired: 1 in, 3 out]
        n221 = Format Into String(format string="AcPwrLoopParameter,%s,%s,-1,%#4g,%#4g,%#4g,%d,#%s", enum16{"AC", "DC"}."DC" ("input 1"), w546, w545, w544, w543, w542, w537) -> (resulting string=w533:string)  [unwired: 2 in, 1 out]
        n222 = invoke class="App" method="Clipboard.Write"("Param 0"=w533) -> ()  [unwired: 3 in, 4 out]
        n223 = Build Array(w533, "Stop" ("element")) -> (w539:string[])
        n224 = call "GetSetTestClass.vi"() -> ("Test.lvclass"=w538:refnum<class "Test.lvclass">)  [unwired: 11 in]
        n225 = call "ScriptedStateMachine.vi"("script"=w539, "Test.lvclass 2"=w538) -> ()  [unwired: 7 in, 3 out]
      }
      event "btnStopParameterLoop": Value Change {
        n226 = event-data() -> ()  [unwired: 1 in, 6 out]
      }
      event Value Change {
        n227 = event-data() -> ()  [unwired: 1 in, 1 out]
        n228 = Unbundle By Name("Loop Parameters") -> ("End Value"=w555:dbl, "Start Value"=w554:dbl, "# Iterations"=w552:u32)
        n229 = Decrement(x=w552) -> (x-1=w549:u32)
        n230 = Subtract(x=w555, y=w554) -> (x-y=w553:dbl)
        n231 = Divide(x=w553, y=w549) -> (x/y=w551:dbl)
        n232 = Bundle By Name(cluster="Loop Parameters", "Increment"=w551) -> (w550:T1)
        n233 = local write "Loop Parameters"(w550) -> ()
      }
      event Value Change {
        n234 = event-data() -> ()  [unwired: 1 in, 1 out]
        n235 = local read "Loop Parameters"() -> (w561:T1)
        n236 = Unbundle By Name(w561) -> ("End Value"=w564:dbl, "Start Value"=w563:dbl, "Increment"=w558:dbl)
        n237 = Subtract(x=w564, y=w563) -> (x-y=w562:dbl)
        n238 = Divide(x=w562, y=w558) -> (x/y=w560:dbl)
        n239 = Round Toward -Infinity(1:w560) -> (0:w557:dbl)
        n240 = Increment(x=w557) -> (x+1=w556:dbl)
        n241 = Bundle By Name(cluster=w561, "# Iterations"=w556) -> (w559:T1)
        n242 = local write "Loop Parameters"(w559) -> ()
      }
      event "ExitHelperLoops?": Value Change {
        n243 = event-data() -> ()  [unwired: 1 in, 1 out]
      }
    }
  }
  n244 = Unregister For Events(event registration refnum=w38) -> (error out=w36:errorcluster)  [unwired: 1 in]
  n245 = flat-sequence {
    tunnel: w10 -> [w567]
    tunnel: w9 -> [_]
    frame #0 {
      n246 = TDMS Close(11:w567) -> ()  [unwired: 1 in, 2 out]
      n247 = property on="ExitHelperLoops?" class="Bool (strict)"("Val(Sgnl)"=TRUE ("Value (Signaling)")) -> ()  [unwired: 2 in, 2 out]
    }
  }
  n248 = flat-sequence {
    tunnel: w36 -> [w571]
    tunnel: [w570] -> w34
    tunnel: w21 -> [w569]
    tunnel: w9 -> [_]
    frame #0 {
      n249 = Release Queue(queue=w569, force destroy? (F)=TRUE, error in (no error)=w571) -> (error out=w570:errorcluster)  [unwired: 2 out]
    }
  }
  n250 = Build Array (concatenate)(w37, w9) -> (w35:errorcluster[])
  n251 = call <userlib>:"AddError.vi"("ErrorArray In"=w35, "error in (no error)"=w34) -> ("ErrorArray Out"=w33:errorcluster[])  [unwired: 8 in, 1 out]
  n252 = disable-structure shown="Disabled" {
    disable-tunnel: w33 -> [w574 w580]
    disable-tunnel: w32 -> [w573 _]
    disable-tunnel: [w572 w580] -> w6
    frame Disabled {
      n253 = Cluster To Array(cluster=w573) -> (array=w575:refnum<user-event>[])
      n254 = for {
        tunnel: w575 -> [w579] mode=indexing
        shift-right: [w578] -> w572
        shift-left: w574 -> [w577]
        n255 = Destroy User Event(user event=w579) -> (error out=w576:errorcluster)  [unwired: 1 in]
        n256 = call <userlib>:"AddError.vi"("ErrorArray In"=w577, "error in (no error)"=w576) -> ("ErrorArray Out"=w578:errorcluster[])  [unwired: 8 in, 1 out]
      }
    }
    frame Enabled {
    }
  }
  "ErrorArray" <- w6
  n257 = Empty Array?(array=w6) -> (empty?=w31:bool)
  n258 = flat-sequence {
    tunnel: "PluginName" -> [w582]
    tunnel: w6 -> [_]
    frame #0 {
      n259 = call "VisDidStop.vi"("DidStop?"=TRUE, "Module Name"=w582) -> ()  [unwired: 9 in, 1 out]
    }
  }
  n260 = case shown="True" w31 {
    tunnel: [w583 _] -> w20
    tunnel: w6 -> [w584 _]
    frame False {
      n261 = Merge Errors(w584) -> (w583:errorcluster)
    }
    frame True {
      n262 = invoke class="VI" method="FP.Close"() -> ()  [unwired: 3 in, 3 out]
    }
  }
  n263 = call <vilib>:"Simple Error Handler.vi"("error in (no error)"=w20) -> ()  [unwired: 4 in, 5 out]
